vi "Get CellFormat.vi"(8 "error in":errorcluster, 10 "Cell In":refnum<k24>, 11 "SpreadsheetDoc in":refnum<k24>) -> (0 "error out":errorcluster, 1 "CellFormat":refnum<k24>, 2 "Cell out":refnum<k24>, 3 "SpreadsheetDoc out":refnum<k24>)   [LabVIEW 2021, in "Open Xml.lvlib"]
uses:
  Open Xml.lvlib
  D:/git/Open-Xml-LabVIEW/dll/DocumentFormat.OpenXml.dll
  dll/DocumentFormat.OpenXml.dll
  D:/git/Open-Xml-LabVIEW/dll/DocumentFormat.OpenXml.Framework.dll
  dll/DocumentFormat.OpenXml.Framework.dll
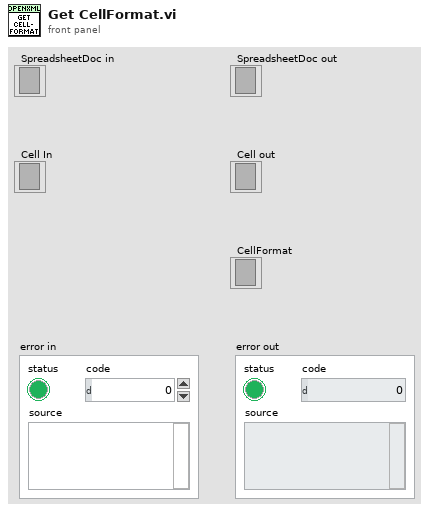
[diagram p1: front panel]
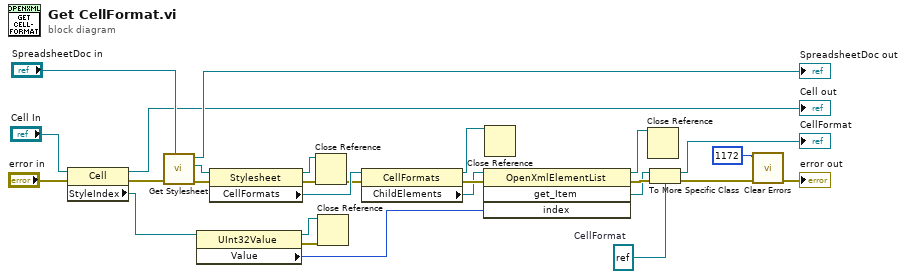
[diagram p0: block diagram]
diagram:
  w23 = refnum<k24> refnum  # CellFormat
  n1 = property class="Cell"(reference="Cell In", error in="error in") -> (reference out=→"Cell out":refnum<k24>, error out=w12:errorcluster, "StyleIndex"=w7:refnum<k24>)
  n2 = call "Get Stylesheet.vi"("error in"=w12, "SpreadsheetDoc in"="SpreadsheetDoc in") -> ("error out"=w17:errorcluster, "Stylesheet"=w10:refnum<k24>, "SpreadsheetDoc out"=→"SpreadsheetDoc out":refnum<k24>)  [unwired: 7 in]
  n3 = property class="UInt32Value"(reference=w7) -> (reference out=w1:refnum<k24>, error out=w2:errorcluster, "Value"=w3:u32)  [unwired: 1 in]
  n4 = property class="Stylesheet"(reference=w10, error in=w17) -> (reference out=w8:refnum<k24>, error out=w20:errorcluster, "CellFormats"=w18:refnum<k24>)
  n5 = Close Reference(reference=w8, error in (no error)=w20) -> (error out=w9:errorcluster)
  n6 = Close Reference(reference=w1, error in (no error)=w2) -> ()  [unwired: 1 out]
  n7 = property class="CellFormats"(reference=w18, error in=w9) -> (reference out=w26:refnum<k24>, error out=w21:errorcluster, "ChildElements"=w19:refnum<k24>)
  n8 = invoke class="OpenXmlElementList" method="get_Item"(reference=w19, error in=w21, "index"=w3) -> (reference out=w27:refnum<k24>, error out=w24:errorcluster, "get_Item"=w22:refnum<k24>)  [unwired: 1 in, 1 out]
  n9 = Close Reference(reference=w26) -> ()  [unwired: 1 in, 1 out]
  n10 = Close Reference(reference=w27) -> ()  [unwired: 1 in, 1 out]
  n11 = To More Specific Class(target class=w23, reference=w22, error in=w24) -> (specific class reference=→"CellFormat":refnum<k24>, error out=w25:errorcluster)
  n12 = call <vilib>:"Clear Errors.vi"("error in (no error)"=w25, "specific error code to clear (0: all)"=1172) -> ("error out"=→"error out":errorcluster)  [unwired: 4 in, 1 out]
